vi "MagX Put File.vi"(6 "timeout (10000)":i32=300000, 8 "error in":errorcluster, 9 "File name":path, 10 "url":string, 11 "client handle":T1) -> (0 "error out":errorcluster, 1 "body":string, 2 "headers":string, 3 "client handle out":T1)   [LabVIEW 2024]
uses:
  <vilib>/httpClient/LabVIEWHTTPClient.lvlib
  <vilib>/httpClient/PUTFile.vi
  <vilib>/httpClient/ClientHandle.ctl
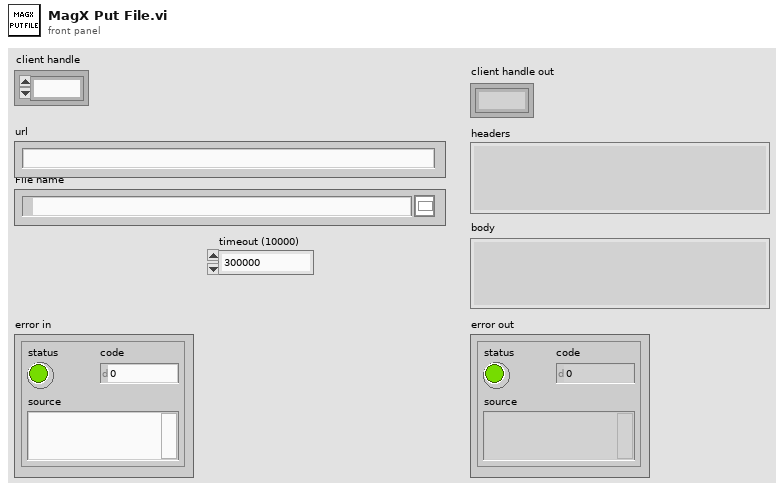
[diagram p1: front panel]
types:
  T1 = typedef "LabVIEWHTTPClient.lvlib/ClientHandle.ctl" = refnum<k1>
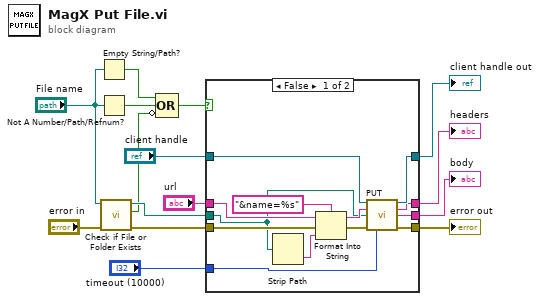
[diagram p0: block diagram]
diagram:
  n1 = Empty String/Path?(string/path="File name") -> (empty?=w4:bool)
  n2 = Not A Number/Path/Refnum?(number/path/refnum="File name") -> (NaN/Path/Refnum?=w3:bool)
  n3 = call <vilib>:"Check if File or Folder Exists.vi"("error in (no error)"="error in", "path"="File name") -> ("error out"=w7:errorcluster, "file or folder exists?"=w1:bool, "dup path"=w6:path)  [unwired: 7 in]
  n4 = Compound Arithmetic op=OR(w4, w3, invert w1) -> (w2:bool)
  n5 = case shown="False" w2 {
    tunnel: "url" -> [w28 _]
    tunnel: "client handle" -> [w26 w30]
    tunnel: [w25 w30] -> w13
    tunnel: [w22 w29] -> w12
    tunnel: [w21 _] -> w11
    tunnel: [w20 _] -> w10
    tunnel: "timeout (10000)" -> [w19 _]
    tunnel: w6 -> [w16 _]
    tunnel: w7 -> [w18 w29]
    frame False {
      n6 = Strip Path(path=w16) -> (name=w17:string)  [unwired: 1 out]
      n7 = Format Into String(format string="&name=%s", initial string=w28, error in=w18, w17) -> (resulting string=w24:string, error out=w23:errorcluster)
      n8 = call-poly <vilib>:"PUT.vi"("client handle"=w26, "url"=w24, "file"=w16, "error in (no error)"=w23, "timeout (10000)"=w19) -> ("client handle out"=w25:T1, "headers"=w20:string, "body"=w21:string, "error out"=w22:errorcluster)  [unwired: 7 in]
    }
    frame True {
    }
  }
  "error out" <- w12
  "client handle out" <- w13
  "body" <- w11
  "headers" <- w10
